vi "Ejemplo1_NumericData.vi"() -> ()   [LabVIEW 2022 SP3]
panel:
  out "x > y?":bool
  in  "Numeric":dbl
  out "Numeric 2":dbl
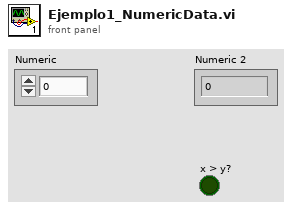
[diagram p1: front panel]
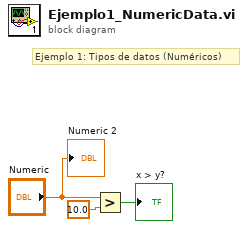
[diagram p0: block diagram]
diagram:
  # "Ejemplo 1: Tipos de datos (Numéricos)"
  n1 = Greater?(x="Numeric", y=10.0) -> (0:→"x > y?":bool)
  "Numeric 2" <- "Numeric"
